vi "5.7-Reliable UPD Client Template.vi"() -> ()   [LabVIEW 2010]
uses:
  6-OCU Neurons/6.0-Super Heart Beat.ctl
  5.0-Global.vi
panel:
  out "Super Heart Beat":T1
  out "My Global Variable":cluster{i32, bool}
  out "Error":errorcluster
  in  "stop":bool
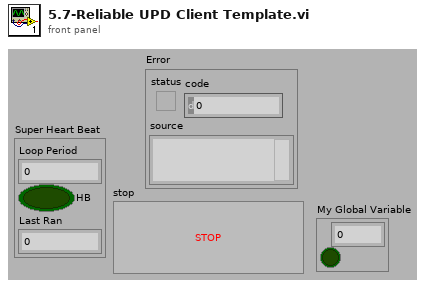
[diagram p1: front panel]
types:
  T1 = typedef "6.0-Super Heart Beat.ctl" = cluster{"Loop Period":u32, "HB":bool, "Last Ran":u32}
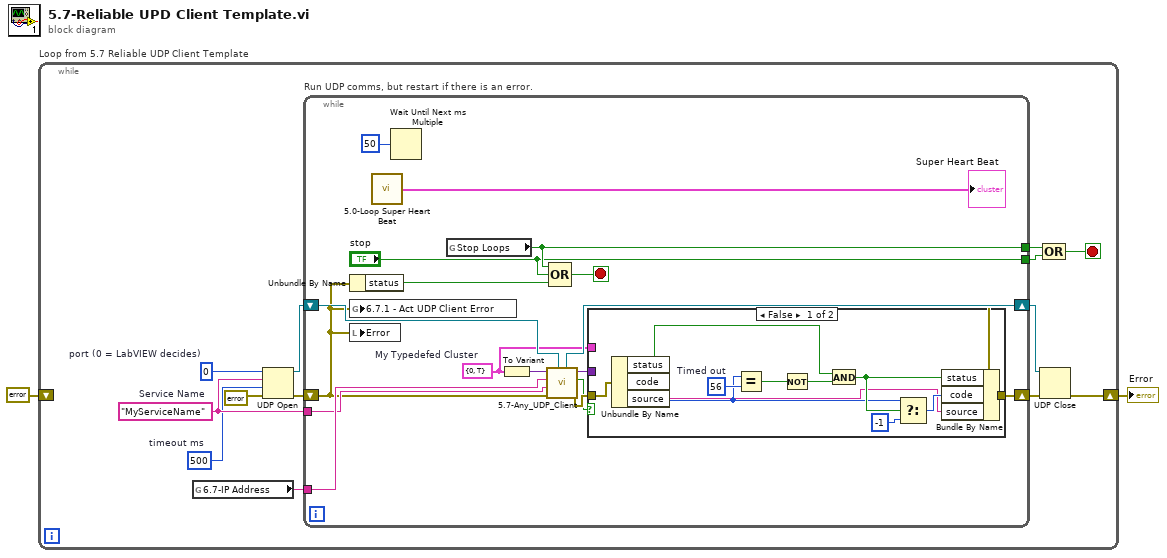
[diagram p0: block diagram]
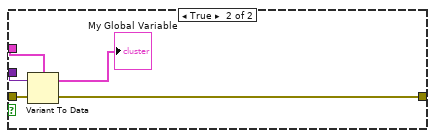
[diagram p2: hidden frame]
diagram:
  n1 = while "Loop from 5.7 Reliable UDP Client Template" {
    shift-right: [w8] -> w2
    shift-left: errorcluster {"status"=FALSE, "code"=0, "source"=""} ("error out") -> [_]
    stop <- w13 stop-if-true
    w5 = 500  # timeout ms
    w7 = u16 0  # port (0 = LabVIEW decides)
    w6 = "MyServiceName"  # Service Name
    n2 = global read "5.0-Global.vi" "6.7-IP Address"() -> (w4:string)
    n3 = UDP Open(8:errorcluster {"status"=FALSE, "code"=0, "source"=""} ("error in (no error)"), 9:w5, 10:w6, 11:w7) -> (port=w12:refnum<k16>, 0:w10:errorcluster)  [unwired: 1 in, 1 out]
    n4 = while "Run UDP comms, but restart if there is an error." {
      tunnel: w6 -> [w29]
      tunnel: w4 -> [w30]
      tunnel: [w26] -> w15
      tunnel: ["stop"] -> w14
      shift-right: [w22] -> w11
      shift-left: w12 -> [w23]
      shift-right: [w21] -> w9
      shift-left: w10 -> [w16]
      stop <- w32 stop-if-true
      w19 = cluster{i32, bool} {0, TRUE}  # My Typedefed Cluster
      n5 = Unbundle By Name(w16) -> ("status"=w24:bool)
      n6 = global write "5.0-Global.vi" "6.7.1 - Act UDP Client Error"(w16) -> ()
      n7 = local write "Error"(w16) -> ()
      n8 = call "5.0-Loop Super Heart Beat.vi"() -> ("Super Heart Beat"=→"Super Heart Beat":T1)
      n9 = Wait Until Next ms Multiple(millisecond multiple=u32 50) -> ()  [unwired: 1 out]
      n10 = global read "5.0-Global.vi" "Stop Loops"() -> (w26:bool)
      n11 = To Variant(anything=w19) -> (Variant=w28:variant)
      n12 = call "5.7-Any_UDP_Client.vi"("Port In"=w23, "error In"=w16, "Service Name"=w29, "IP Address"=w30, "DataTypeIn"=w28) -> ("Error Out"=w20:errorcluster, "Check Passed"=w18:bool, "DataOut"=w27:variant, "Port out"=w22:refnum<k16>)  [unwired: 3 in]
      n13 = Compound Arithmetic op=OR(w26, "stop", w24) -> (w32:bool)
      n14 = case "Ignore Timeouts" shown="False" w18 {
        tunnel: w27 -> [_ w48]
        tunnel: w19 -> [_ w47]
        tunnel: w20 -> [w43 w46]
        tunnel: [w42 w45] -> w21
        frame False {
          w41 = 56  # Timed out
          n15 = Unbundle By Name(w43) -> ("status"=w38:bool, "code"=w36:i32, "source"=w33:string)
          n16 = Equal?(x=w36, y=w41) -> (x = y?=w40:bool)
          n17 = Not(x=w40) -> (.not. x?=w39:bool)
          n18 = And(x=w38, y=w39) -> (x .and. y?=w37:bool)
          n19 = Select(t=w36, s=w37, f=-1) -> (s? t:f=w34:i32)
          n20 = Bundle By Name(cluster=w43, "status"=w37, "code"=w34, "source"=w33) -> (w42:errorcluster)
        }
        frame True {
          n21 = Variant To Data(error in=w46, Variant=w48, type=w47) -> (error out=w45:errorcluster, data=→"My Global Variable":cluster{i32, bool})
        }
      }
    }
    n22 = UDP Close(connection ID=w11, 8:w9) -> (error out=w8:errorcluster)  [unwired: 1 out]
    n23 = Compound Arithmetic op=OR(w15, w14) -> (w13:bool)
  }
  "Error" <- w2
